vi "Save images.vi"() -> ()   [LabVIEW 2013]
panel:
  in  "Cancel Button":bool
  in  "address":string="192.168.0.90"
  out "Image":T1(plugin-control)
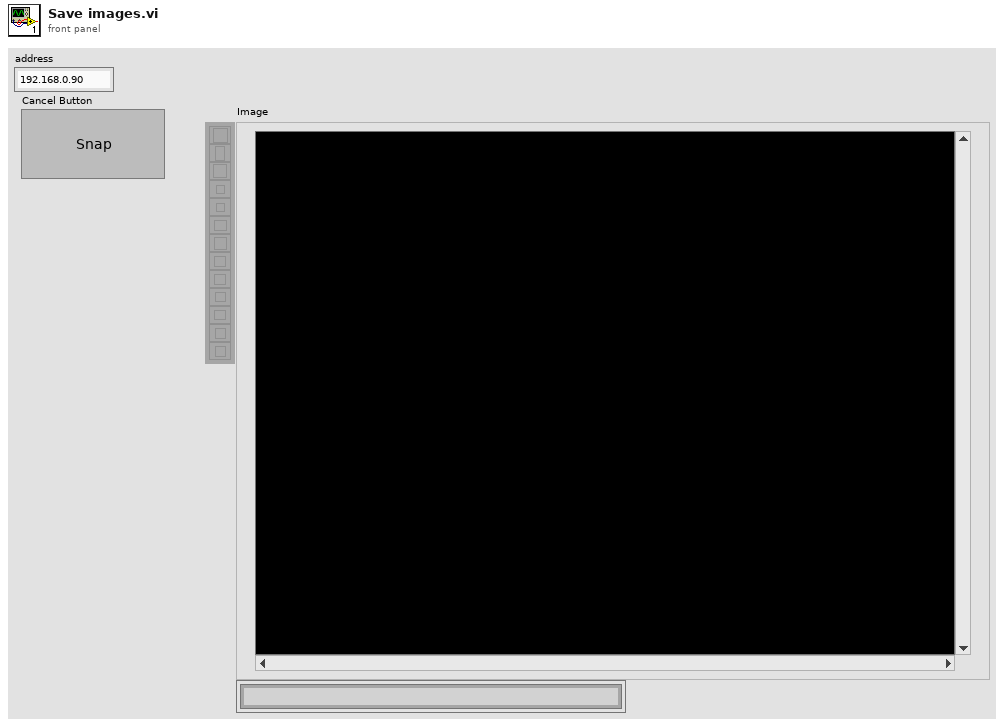
[diagram p1: front panel]
types:
  T1 = typedef "IMAQ Image.ctl" = refnum<image>
  T2 = typedef "Image Type" = u32
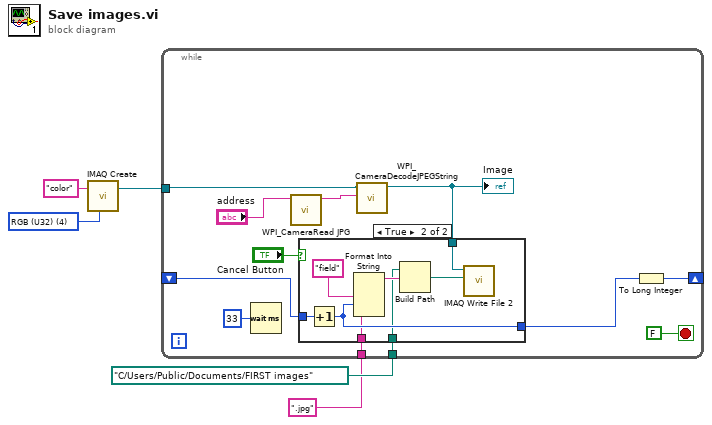
[diagram p0: block diagram]
diagram:
  w4 = T2 4 items=["Grayscale (U8)", "Grayscale (I16)", "Grayscale (SGL)", "Complex (CSG)", "RGB (U32)", "HSL (U32)", "RGB (U64)", "Grayscale (U16)"] ("Image Type")
  n1 = call "IMAQ Create"("Image Name"="color", "Image Type"=w4) -> ("New Image"=w3:T1)  [unwired: 3 in, 1 out]
  n2 = while {
    tunnel: w3 -> [w16]
    shift-right: [w7] -> _
    shift-left: _ -> [w12]
    tunnel: path "C:/Users/Public/Documents/FIRST images" -> [w10]
    tunnel: ".jpg" -> [w6]
    stop <- FALSE stop-if-true
    n3 = Wait (ms)(milliseconds to wait=u32 33) -> ()  [unwired: 1 out]
    n4 = call <vilib>:"WPI_CameraRead JPG.vi"("address"="address") -> ("Raw Image Data"=w17:string)  [unwired: 9 in, 1 out]
    n5 = call <vilib>:"WPI_CameraDecodeJPEGString.vi"("Compressed Image"=w17, "Image In"=w16) -> ("Image Out"=w9:T1)  [unwired: 4 in, 1 out]
    "Image" <- w9
    n6 = case shown="True" "Cancel Button" {
      tunnel: w12 -> [w18 w26]
      tunnel: [w18 w25] -> w11
      tunnel: w10 -> [_ w23]
      tunnel: w9 -> [_ w21]
      tunnel: w6 -> [_ w19]
      frame False {
      }
      frame True {
        n7 = Increment(x=w26) -> (x+1=w25:i32)
        n8 = Format Into String("field", w25, w19) -> (resulting string=w24:string)  [unwired: 3 in, 1 out]
        n9 = Build Path(base path=w23, name or relative path=w24) -> (appended path=w22:path)
        n10 = call-poly "IMAQ Write File 2"("File Path"=w22, "Image"=w21) -> ()  [unwired: 8 in, 2 out]
      }
    }
    n11 = To Long Integer(number=w11) -> (32bit integer=w7:i32)
  }
